vi "Search Current.vi"(5 "BoardHandle in":T1, 7 "Channel # in":i32, 11 "error in (no error)":errorcluster, 12 "Stop Program Search Current":bool) -> (1 "Actual Voltage Level (V)":dbl format="%#_13g", 2 "Power Supply Trip":bool, 3 "Actual Current Limit (nA)":dbl format="%#_13g", 10 "Array":dbl[](array[numeric]), 14 "BoardHandle out 2":T1, 15 "error out":errorcluster)   [LabVIEW 2020]
uses:
  Program Files/National Instruments/LabVIEW 2018/instr.lib/CAEN PSM/CAEN PSM.lvlib
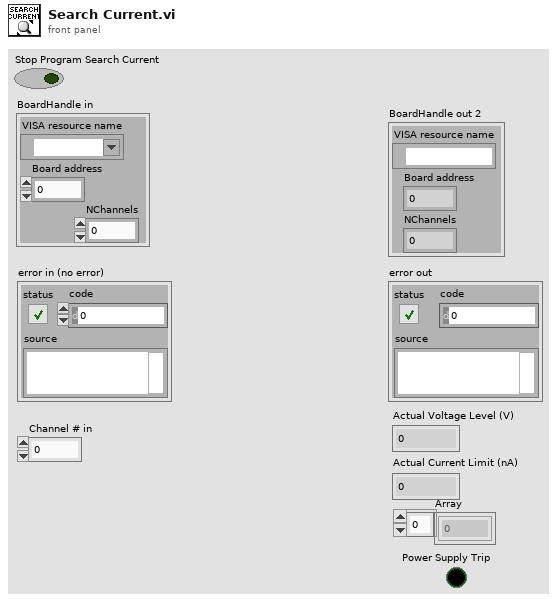
[diagram p1: front panel]
types:
  T1 = cluster{"VISA resource name":refnum<visa-resource-name>, "Board address":u8, "NChannels":u8}
  T2 = typedef "CAEN PSM.lvlib/BoardHandle.ctl" = cluster{"VISA resource name":refnum<visa-resource-name>, "Board address":u8, "NChannels":u8}
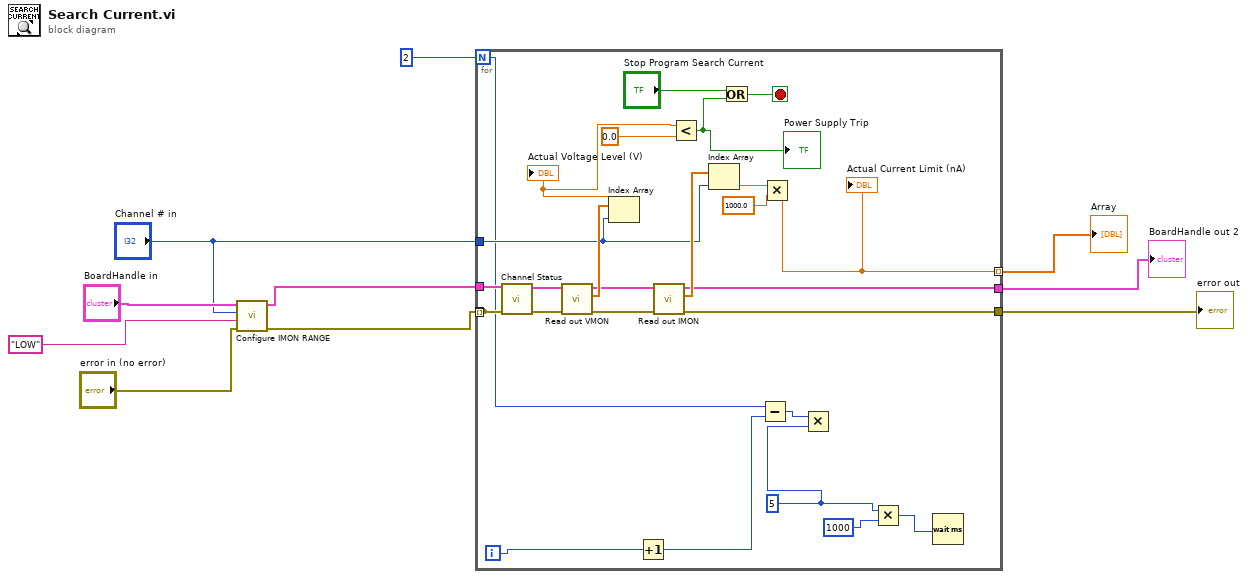
[diagram p0: block diagram]
diagram:
  n1 = call "Configure IMON RANGE.vi"("error in (no error)"="error in (no error)", "IMon range (LOW)"="LOW", "Channel (0)"="Channel # in", "BoardHandle"="BoardHandle in") -> ("error out"=w4:errorcluster, "BoardHandle out"=w5:T2)  [unwired: 6 in]
  n2 = for {
    N: 2 ("N") -> [w20]
    tunnel: w4 -> [w27]
    tunnel: "Channel # in" -> [w28]
    tunnel: [w30] -> w8
    tunnel: [w29] -> w9
    tunnel: [w21] -> w10 mode=indexing
    tunnel: w5 -> [w24]
    tunnel: [w27] -> _ mode=indexing
    i -> [w18]
    stop <- w13 stop-if-true
    w14 = 5 ("dt (s) in")
    n3 = call "Channel Status.vi"("error in (no error)"=w27, "BoardHandle"=w24) -> ("error out"=w36:errorcluster, "BoardHandle out"=w35:T2)  [unwired: 7 in, 1 out]
    n4 = call "Read out VMON.vi"("error in (no error)"=w36, "BoardHandle"=w35) -> ("error out"=w32:errorcluster, "VMon values (V)"=w34:dbl[], "BoardHandle out"=w33:T2)  [unwired: 7 in]
    n5 = Index Array(array=w34, index=w28) -> (element=w16:dbl)
    "Actual Voltage Level (V)" <- w16
    n6 = Increment(x=w18) -> (x+1=w17:i32)
    n7 = call "Read out IMON.vi"("error in (no error)"=w32, "BoardHandle"=w33) -> ("error out"=w29:errorcluster, "IMon values (uA)"=w31:dbl[], "BoardHandle out"=w30:T2)  [unwired: 6 in, 1 out]
    n8 = Less?(x=w16, y=0.0) -> (x < y?=w12:bool)
    "Power Supply Trip" <- w12
    n9 = Index Array(array=w31, index=w28) -> (element=w23:dbl)
    n10 = Or(x="Stop Program Search Current", y=w12) -> (x .or. y?=w13:bool)
    n11 = Subtract(x=w20, y=w17) -> (x-y=w19:i32)
    n12 = Multiply(x=w23, y=1000.0) -> (x*y=w21:dbl)
    "Actual Current Limit (nA)" <- w21
    n13 = Multiply(x=w19, y=w14) -> ()  [unwired: 1 out]
    n14 = Multiply(x=w14, y=1000) -> (x*y=w26:i32)
    n15 = Wait (ms)(milliseconds to wait=w26) -> ()  [unwired: 1 out]
  }
  "Array" <- w10
  "error out" <- w9
  "BoardHandle out 2" <- w8
